vi "Find control by label.vi"(8 "error in (no error)":errorcluster, 10 "Label":string="Parameters", 11 "VI ref":refnum<vi>) -> (0 "error out":errorcluster, 2 "Found":bool, 3 "Control out":refnum<vi>)   [LabVIEW 2015]
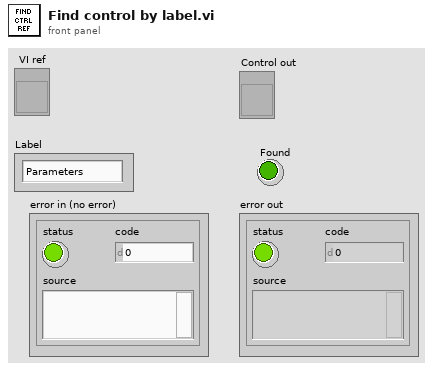
[diagram p1: front panel]
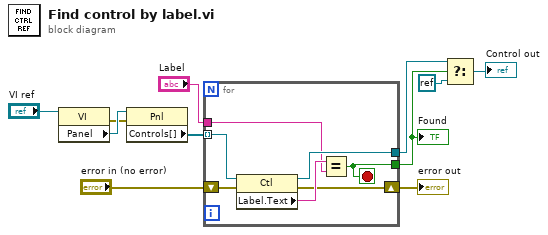
[diagram p0: block diagram]
diagram:
  n1 = property class="VI"(reference="VI ref") -> (error out=w7:errorcluster, "Panel"=w8:refnum<vi>)  [unwired: 1 in, 1 out]
  n2 = property class="Pnl"(reference=w8, error in=w7) -> ("Controls[]"=w5:refnum<vi>[])  [unwired: 2 out]
  n3 = for {
    tunnel: w5 -> [w17] mode=indexing
    tunnel: [w15] -> w4
    tunnel: [w14] -> w3
    shift-right: [w13] -> w11
    shift-left: "error in (no error)" -> [w18]
    tunnel: "Label" -> [w12]
    stop <- w15 stop-if-true
    n4 = property class="Ctl"(reference=w17, error in=w18) -> (reference out=w14:refnum<vi>, error out=w13:errorcluster, "Label.Text"=w16:string)
    n5 = Equal?(x=w16, y=w12) -> (x = y?=w15:bool)
  }
  "Found" <- w4
  "error out" <- w11
  n6 = Select(t=w3, s=w4, f=refnum<k0> refnum) -> (s? t:f=→"Control out":refnum<vi>)
